vi "Increment ID.vi"(8 "error in (no error)":errorcluster, 11 "Panel Actor With Events in":refnum<class "Helper Methods.lvclass">) -> (0 "error out":errorcluster, 3 "Panel Actor With Events out":refnum<class "Helper Methods.lvclass">)   [LabVIEW 2020, in "2. Basic Panel Actors.lvlib" / "Helper Methods.lvclass"]
uses:
  Helper Methods.lvclass
  Helper Methods.lvclass/Helper Methods.ctl
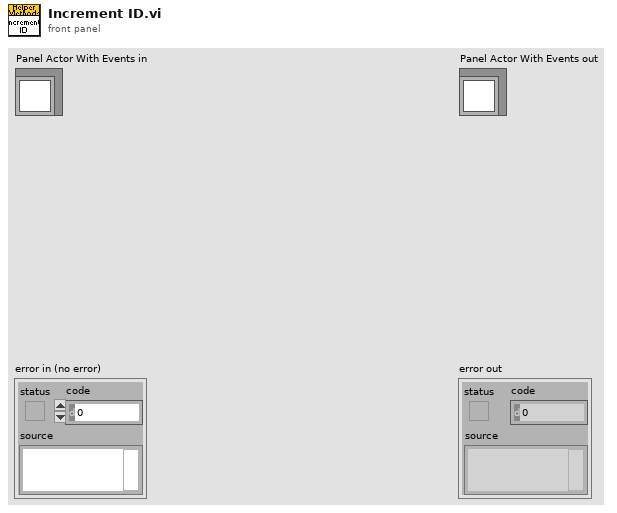
[diagram p1: front panel]
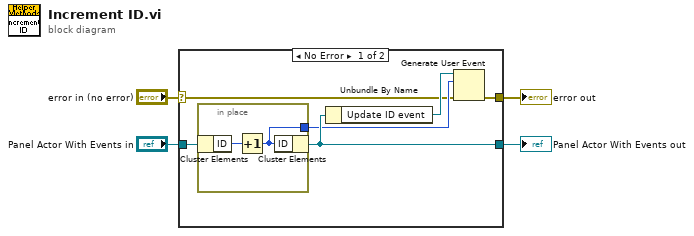
[diagram p0: block diagram]
diagram:
  n1 = case shown="No Error" "error in (no error)" {
    selector: "error in (no error)" -> [w6 w14]
    tunnel: [w5 w14] -> w3
    tunnel: [w9 w13] -> w1
    tunnel: "Panel Actor With Events in" -> [w10 w13]
    frame No Error {
      n2 = in-place {
        in-place-border: [w11] -> w7
        n3 = in-place-cluster #1(w10) -> ("ID"=w12:i32)
        n4 = Increment(x=w12) -> (x+1=w11:i32)
        n5 = in-place-cluster #1("ID"=w11) -> (w9:refnum<class "Helper Methods.lvclass">)
      }
      n6 = Unbundle By Name(w9) -> ("Update ID event"=w8:refnum<user-event>)
      n7 = Generate User Event(user event=w8, event data cluster=w7, error in=w6) -> (error out=w5:errorcluster)  [unwired: 1 in, 1 out]
    }
    frame Error {
    }
  }
  "error out" <- w3
  "Panel Actor With Events out" <- w1
